vi "TTA_Write_Test_List.vi"() -> ()   [LabVIEW 2016]
uses:
  <vilib>/Utility/config.llb/Write Key (String).vi
  <vilib>/Utility/config.llb/NI_LVConfig.lvlib
panel:
  in  "Rx Test List":string[](array[string])=["Received_Power", "Phase", "ACPR"]
  in  "Tx Test List":string[](array[string])=["Output_Power", "Phase", "ACPR", "Set_Power_Cal"]
  in  "RFIC Test List":string[](array[string])=["Software_Version_&_Update_Test", "MP_Loop_Back_Test", "Download_PAL_Firmware", "Digital_SPI_Test", "RFIC_Initialization", "PLL_Lock", "RFIC_BDS_Tone_Test", "RFIC_Temperature_Test", "Set_Digital_Attenuation", "PAL_Linearization", "Tx_RFCAL_Diagnostics", "Rx_RFCAL_Diagnostics"]
  in  "error in (no error)":errorcluster
  in  "Working Directory":path
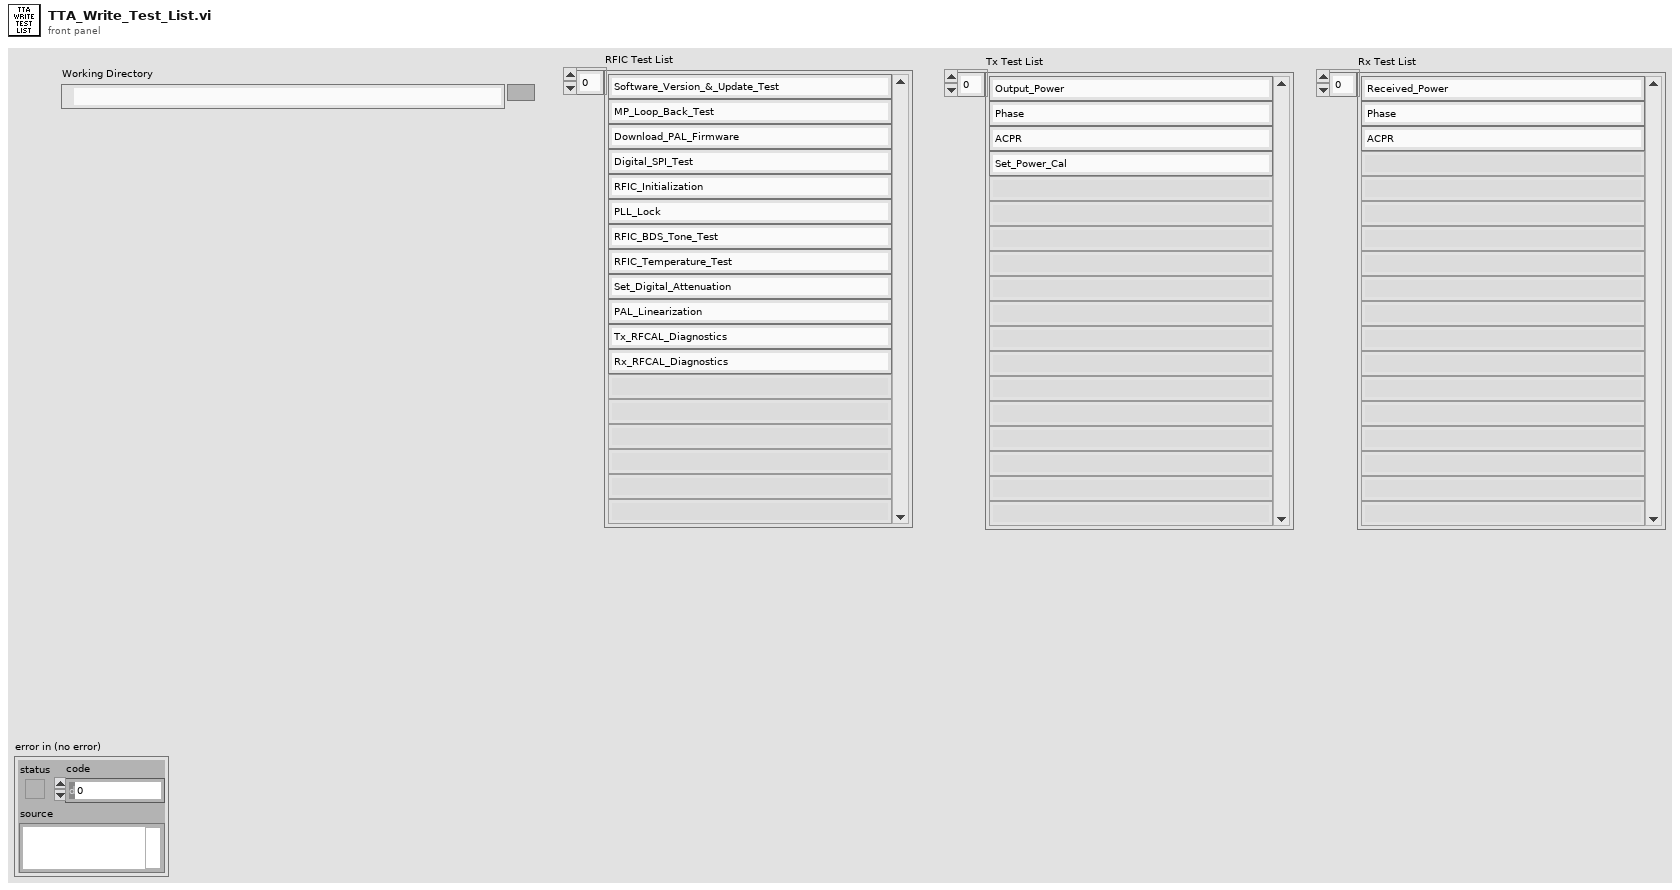
[diagram p1: front panel]
types:
  T1 = typedef "NI_LVConfig.lvlib/Config Data RefNum.ctl" = refnum<k1>
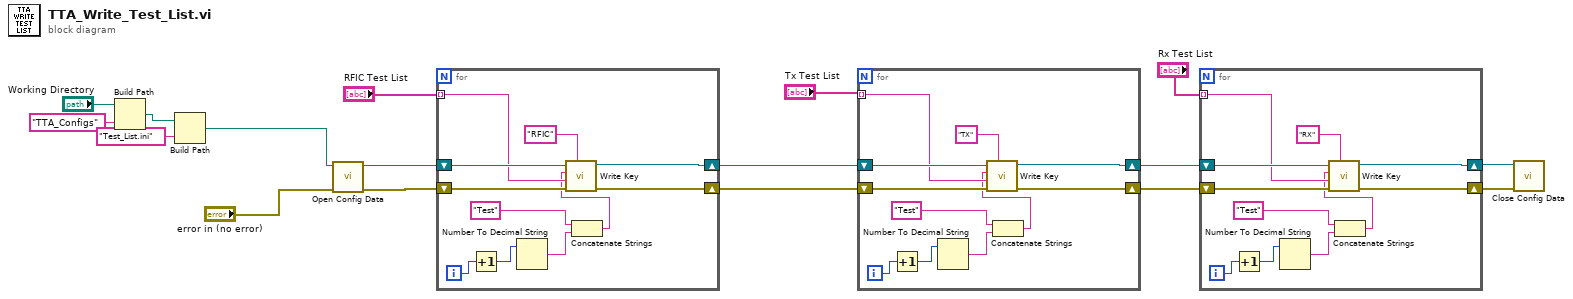
[diagram p0: block diagram]
diagram:
  n1 = Build Path(base path="Working Directory", name or relative path="TTA_Configs") -> (appended path=w3:path)
  n2 = Build Path(base path=w3, name or relative path="Test_List.ini") -> (appended path=w1:path)
  n3 = call <vilib>:"Open Config Data.vi"("error in (no error)"="error in (no error)", "configuration file path"=w1) -> ("error out"=w15:errorcluster, "refnum"=w16:T1)  [unwired: 7 in, 1 out]
  n4 = for {
    shift-right: [w26] -> w11
    shift-left: w15 -> [w25]
    shift-right: [w24] -> w12
    shift-left: w16 -> [w28]
    tunnel: "RFIC Test List" -> [w23] mode=indexing
    i -> [w22]
    n5 = Increment(x=w22) -> (x+1=w21:i32)
    n6 = Number To Decimal String(number=w21) -> (decimal integer string=w20:string)  [unwired: 1 in]
    n7 = Concatenate Strings("Test" ("key"), w20) -> (w18:string)
    n8 = call-poly <vilib>:"Write Key.vi"("section"="RFIC", "error in (no error)"=w25, "value"=w23, "key"=w18, "refnum"=w28) -> ("error out"=w26:errorcluster, "refnum out"=w24:T1)  [unwired: 4 in, 1 out]
  }
  n9 = for {
    shift-right: [w37] -> w10
    shift-left: w11 -> [w36]
    shift-right: [w35] -> w9
    shift-left: w12 -> [w39]
    tunnel: "Tx Test List" -> [w34] mode=indexing
    i -> [w33]
    n10 = Increment(x=w33) -> (x+1=w32:i32)
    n11 = Number To Decimal String(number=w32) -> (decimal integer string=w31:string)  [unwired: 1 in]
    n12 = Concatenate Strings("Test" ("key"), w31) -> (w29:string)
    n13 = call-poly <vilib>:"Write Key.vi"("section"="TX", "error in (no error)"=w36, "value"=w34, "key"=w29, "refnum"=w39) -> ("error out"=w37:errorcluster, "refnum out"=w35:T1)  [unwired: 4 in, 1 out]
  }
  n14 = for {
    shift-right: [w48] -> w7
    shift-left: w10 -> [w47]
    shift-right: [w46] -> w6
    shift-left: w9 -> [w50]
    tunnel: "Rx Test List" -> [w45] mode=indexing
    i -> [w44]
    n15 = Increment(x=w44) -> (x+1=w43:i32)
    n16 = Number To Decimal String(number=w43) -> (decimal integer string=w42:string)  [unwired: 1 in]
    n17 = Concatenate Strings("Test" ("key"), w42) -> (w40:string)
    n18 = call-poly <vilib>:"Write Key.vi"("section"="RX", "error in (no error)"=w47, "value"=w45, "key"=w40, "refnum"=w50) -> ("error out"=w48:errorcluster, "refnum out"=w46:T1)  [unwired: 4 in, 1 out]
  }
  n19 = call <vilib>:"Close Config Data.vi"("error in (no error)"=w7, "refnum"=w6) -> ()  [unwired: 8 in, 2 out]
